vi "Insert Group Create Params.vi"(8 "error in":errorcluster, 11 "TDMS in":refnum<class "TDMS.lvclass">) -> (0 "error out":errorcluster, 3 "TDMS out":refnum<class "TDMS.lvclass">)   [LabVIEW 2019, in "TDMS.lvlib" / "TDMS.lvclass"]
uses:
  TDMS.lvclass
  TDMS.lvclass/TDMS.ctl
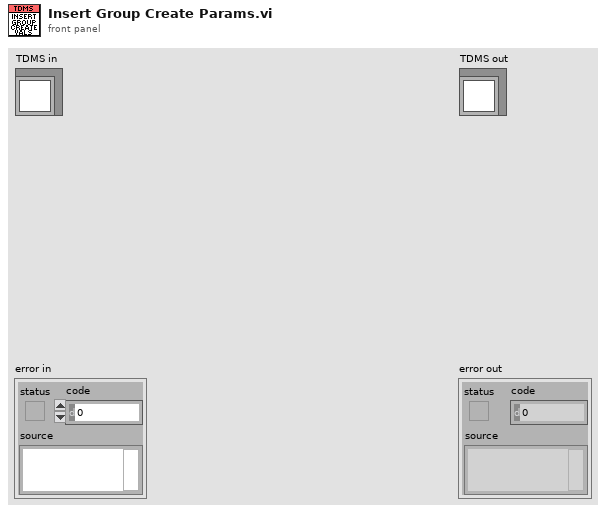
[diagram p1: front panel]
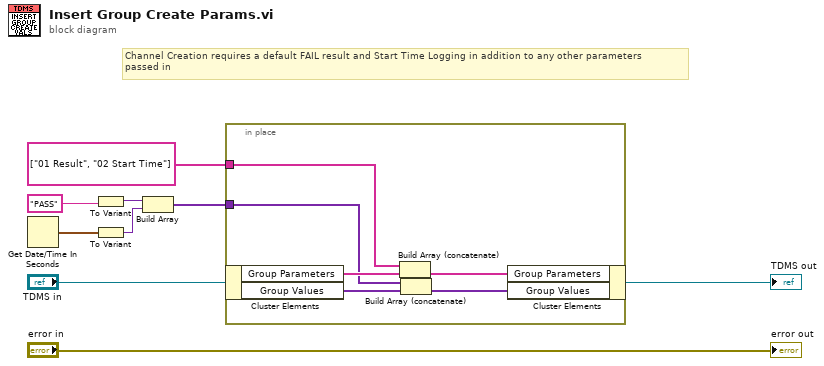
[diagram p0: block diagram]
diagram:
  # "Channel Creation requires a default FAIL result and Start Time Logging in addition to any other parameters \npassed in"
  n1 = Get Date/Time In Seconds() -> (seconds since 1Jan1904=w9:timestamp)
  n2 = To Variant(anything="PASS") -> (Variant=w5:variant)
  n3 = To Variant(anything=w9) -> (Variant=w4:variant)
  n4 = Build Array(w5, w4) -> (w3:variant[])
  n5 = in-place {
    in-place-border: string[] ["01 Result", "02 Start Time"] -> [w13]
    in-place-border: w3 -> [w10]
    n6 = in-place-cluster #1("TDMS in") -> ("Group Parameters"=w15:string[], "Group Values"=w12:variant[])
    n7 = Build Array (concatenate)(w13, w15) -> (w14:string[])
    n8 = Build Array (concatenate)(w10, w12) -> (w11:variant[])
    n9 = in-place-cluster #1("Group Parameters"=w14, "Group Values"=w11) -> (→"TDMS out":refnum<class "TDMS.lvclass">)
  }
  "error out" <- "error in"
